vi "GetPMUNumber.vi"(8 "error in (no error)":errorcluster, 11 "Accessors:clEvtReportArray":T1 {"Synx" format="%#_4g"}) -> (0 "error out":errorcluster, 3 "size(s)":i32)   [LabVIEW 2017, in "AppPlugins.lvlib" / "LSEPlugin.lvclass"]
uses:
  LSEPlugin.lvclass
  EventPlugins/EventPluginBaseClass/TypeDefs/clEvtReportArray.ctl
  EventPlugins/EventPluginBaseClass/TypeDefs/clEvtReport.ctl
  EventPlugins/EventPluginBaseClass/EventPluginBaseClass.lvclass
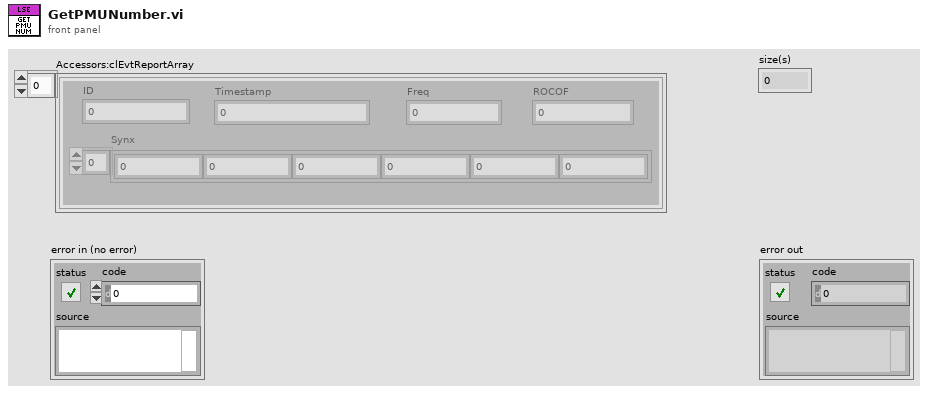
[diagram p1: front panel]
types:
  T1 = typedef "EventPlugins.lvlib/EventPluginBaseClass.lvclass/clEvtReportArray.ctl" = T2[]
  T2 = typedef "EventPlugins.lvlib/EventPluginBaseClass.lvclass/clEvtReport.ctl" = cluster{"Timestamp":dbl, "Synx":cdb[], "Freq":dbl, "ROCOF":dbl, "ID":i16}
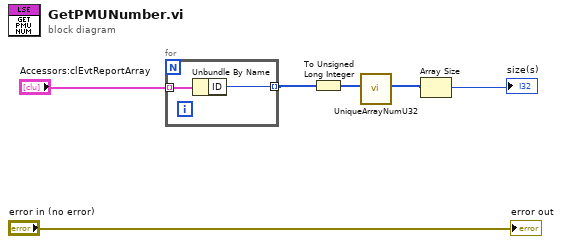
[diagram p0: block diagram]
diagram:
  n1 = for {
    tunnel: "Accessors:clEvtReportArray" -> [w8] mode=indexing
    tunnel: [w7] -> w3 mode=indexing
    n2 = Unbundle By Name(w8) -> ("ID"=w7:i16)
  }
  n3 = To Unsigned Long Integer(number=w3) -> (unsigned 32bit integer=w6:u32[])
  n4 = call "UniqueArrayNumU32.vi"("Input Array"=w6) -> ("Output Array"=w2:u32[])  [unwired: 8 in]
  n5 = Array Size(array=w2) -> (size(s)=→"size(s)":i32)
  "error out" <- "error in (no error)"
